vi "ReadParams.vi"() -> (0 "Force RY":dbl, 1 "Force RX":dbl, 2 "Force LY":dbl, 3 "Force LX":dbl, 4 "Left Pot Gradient":dbl, 5 "Right Pot Offset":dbl, 6 "Left Pot Offset":dbl, 7 "Right Pot Gradient":dbl)   [LabVIEW 2019]
uses:
  <vilib>/Utility/file.llb/Read Delimited Spreadsheet (DBL).vi
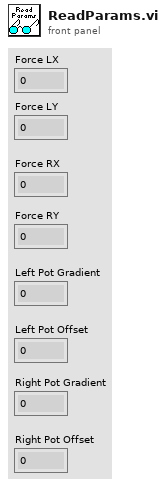
[diagram p1: front panel]
types:
  T1 = cluster{"all rows[0]":dbl, "all rows[1]":dbl, "all rows[2]":dbl, "all rows[3]":dbl, "all rows[4]":dbl, "all rows[5]":dbl, "all rows[6]":dbl, "all rows[7]":dbl, "all rows[8]":dbl}
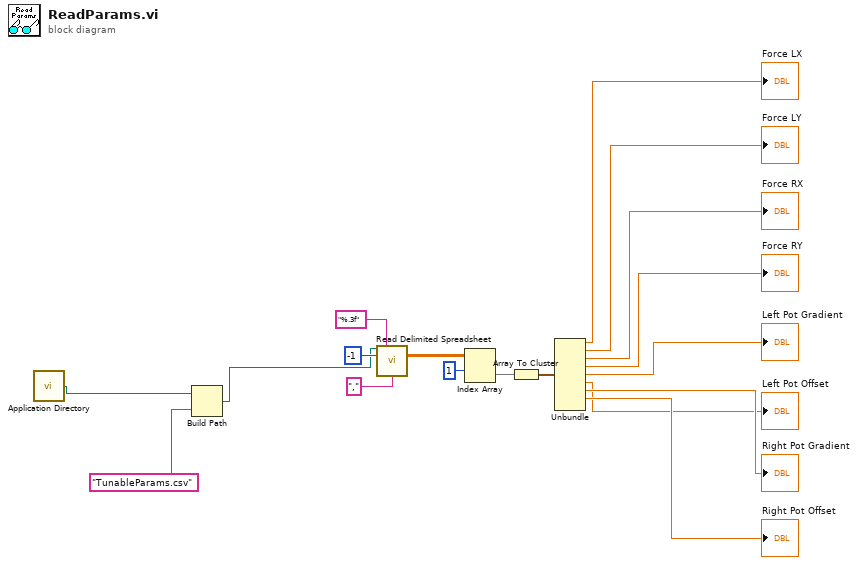
[diagram p0: block diagram]
diagram:
  n1 = call <vilib>:"Application Directory.vi"() -> ("Application Directory"=w2:path)
  n2 = Build Path(base path=w2, name or relative path="TunableParams.csv") -> (appended path=w3:path)
  n3 = call-poly <vilib>:"Read Delimited Spreadsheet.vi"("file path (dialog if empty)"=w3, "format (%.3f)"="%.3f", "number of rows (all:-1)"=-1, "delimiter (\\t)"="," ("delimiter (\\t)")) -> ("all rows"=w7:dbl[][])  [unwired: 6 in, 5 out]
  n4 = Index Array(array=w7, index (row)=1) -> (element=w9:dbl[])  [unwired: 1 in]
  n5 = Array To Cluster(array=w9) -> (cluster=w10:T1)
  n6 = Unbundle(w10) -> ("all rows[0]"=→"Force LX":dbl, "all rows[1]"=→"Force LY":dbl, "all rows[2]"=→"Force RX":dbl, "all rows[3]"=→"Force RY":dbl, "all rows[4]"=→"Left Pot Gradient":dbl, "all rows[5]"=→"Left Pot Offset":dbl, "all rows[6]"=→"Right Pot Gradient":dbl, "all rows[7]"=→"Right Pot Offset":dbl)  [unwired: 1 out]
